vi "2022 Create Winch Constants.vi"(8 "error in (no error)":errorcluster, 10 "localConstantSpreadSheet":string[][](array[string]), 11 "robotID":string) -> (0 "error out":errorcluster)   [LabVIEW 2020]
uses:
  2022 Robot Global Data.vi
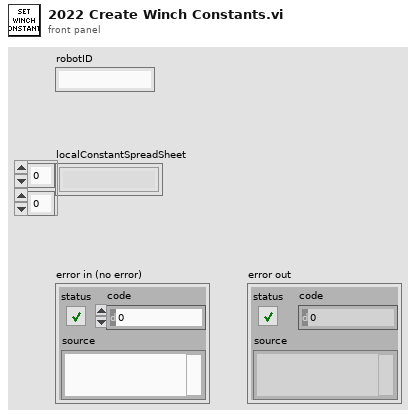
[diagram p1: front panel]
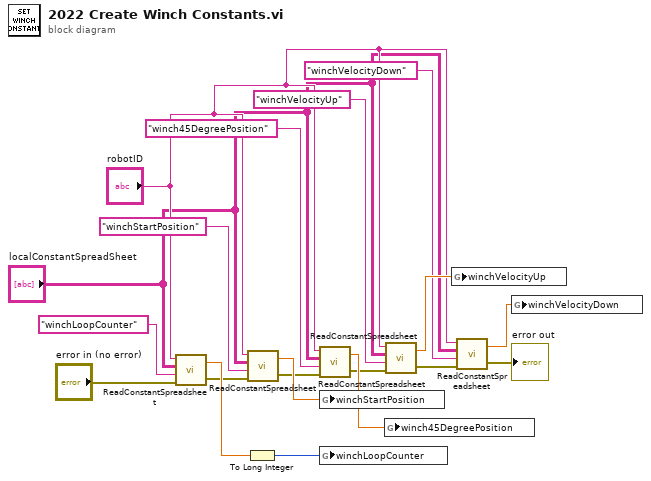
[diagram p0: block diagram]
diagram:
  n1 = call "ReadConstantSpreadsheet.vi"("error in"="error in (no error)", "Constant"="winchLoopCounter", "2022ConstantSpreadSheet"="localConstantSpreadSheet", "Robot ID"="robotID") -> ("error out"=w5:errorcluster, "Constant Value"=w15:dbl)
  n2 = To Long Integer(number=w15) -> (32bit integer=w16:i32)
  n3 = call "ReadConstantSpreadsheet.vi"("error in"=w5, "Constant"="winchStartPosition", "2022ConstantSpreadSheet"="localConstantSpreadSheet", "Robot ID"="robotID") -> ("error out"=w4:errorcluster, "Constant Value"=w19:dbl)
  n4 = call "ReadConstantSpreadsheet.vi"("error in"=w4, "Constant"="winch45DegreePosition", "2022ConstantSpreadSheet"="localConstantSpreadSheet", "Robot ID"="robotID") -> ("error out"=w3:errorcluster, "Constant Value"=w13:dbl)
  n5 = global write "2022 Robot Global Data.vi" "winchStartPosition"(w19) -> ()
  n6 = global write "2022 Robot Global Data.vi" "winchLoopCounter"(w16) -> ()
  n7 = global write "2022 Robot Global Data.vi" "winch45DegreePosition"(w13) -> ()
  n8 = call "ReadConstantSpreadsheet.vi"("error in"=w3, "Constant"="winchVelocityUp", "2022ConstantSpreadSheet"="localConstantSpreadSheet", "Robot ID"="robotID") -> ("error out"=w2:errorcluster, "Constant Value"=w11:dbl)
  n9 = global write "2022 Robot Global Data.vi" "winchVelocityUp"(w11) -> ()
  n10 = call "ReadConstantSpreadsheet.vi"("error in"=w2, "Constant"="winchVelocityDown", "2022ConstantSpreadSheet"="localConstantSpreadSheet", "Robot ID"="robotID") -> ("error out"=→"error out":errorcluster, "Constant Value"=w9:dbl)
  n11 = global write "2022 Robot Global Data.vi" "winchVelocityDown"(w9) -> ()
